vi "Get VISA resource name.vi"(11 "DAM0404D in":refnum<class "DAM0404D.lvclass">) -> (2 "VISA resource name":refnum<vi>, 3 "DAM0404D out":refnum<class "DAM0404D.lvclass">)   [LabVIEW 2016, in "DAM0404D.lvlib" / "DAM0404D.lvclass"]
uses:
  DAM0404D.lvclass
  DAM0404D.lvclass/DAM0404D.ctl
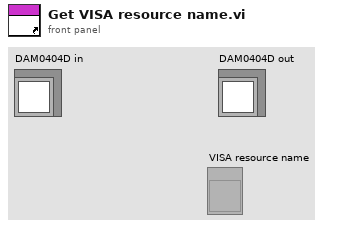
[diagram p1: front panel]
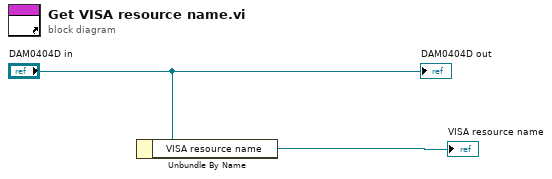
[diagram p0: block diagram]
diagram:
  n1 = Unbundle By Name("DAM0404D in") -> ("VISA resource name"=→"VISA resource name":refnum<vi>)
  "DAM0404D out" <- "DAM0404D in"
